vi "configure.vi"(8 "error in (no error)":errorcluster, 11 "DL090623TwoDAnalyser in":refnum<class "AnalyserDL090623TwoD.lvclass">) -> (0 "error out":errorcluster, 3 "DL090623TwoDAnalyser out":refnum<class "AnalyserDL090623TwoD.lvclass">)   [LabVIEW 2010, in "AnalyserDL090623TwoD.lvclass"]
doc: "The dynamic dispatch version of this VI loads and displays the configuration file associated with the plug-in object. The user modify and save the configuration data."
uses:
  AnalyserDL090623TwoD.lvclass
  common/xcontrols/XComponentSpecification/XComponentSpecification/XComponentSpecification.xctl
  AnalyserDL090623TwoD.lvclass/AnalyserDL090623TwoD.ctl
  Segmenter/GenericSegmenter/GenericSegmenter/GenericSegmenter.lvclass
  TraceProcessor/GenericTraceProcessor/GenericTraceProcessor/GenericTraceProcessor.lvclass
  common/classes/ErrorController/ErrorController/class_data.vi
  common/classes/GenericComponent/GenericComponent/GenericComponent.lvclass
  common/classes/ErrorController/ErrorController/ErrorController.lvclass
panel:
  in  "segmenter spec":T1(xcontrol)
  out "Configuration":string
  in  "Tab Control":T2(tab)
  in  "channel calculation expression":string
  in  "configure trace processors":bool
  in  "cancel button":bool
  in  "save button":bool
  # "Configure AnalyserDL090623TwoD"
  # "The AnalyserDL090623TwoD component receives images and calculates the mean signal intensity on image ROIs according to an arithmetic expression (see trace specification). \nROIs can either be drawn by hand and automatically determined using a Segmenter. \nThese intensity values are sent through a pipeline of TraceProcessors, which can perform further mathematic analysis on them."
  # "This mathematic term specifies how traces are calculated from channels. Enter an expression containing the channels as capital letters in alphabetic order. \nIMPORTANT: Numeric constants are not yet supported.\n\n \n- if you want to refer to the second channel only: B\n- if you want to refer to the ratio of the second and third channel: B/C\n- more complicated example: (A-B)/C+D"
  # "Traces calculated from the channels based on the trace specification expression given on the previous tab are processed by a user-defined pipeline of TraceProcessors. Each TraceProcessor may have a display to show its result."
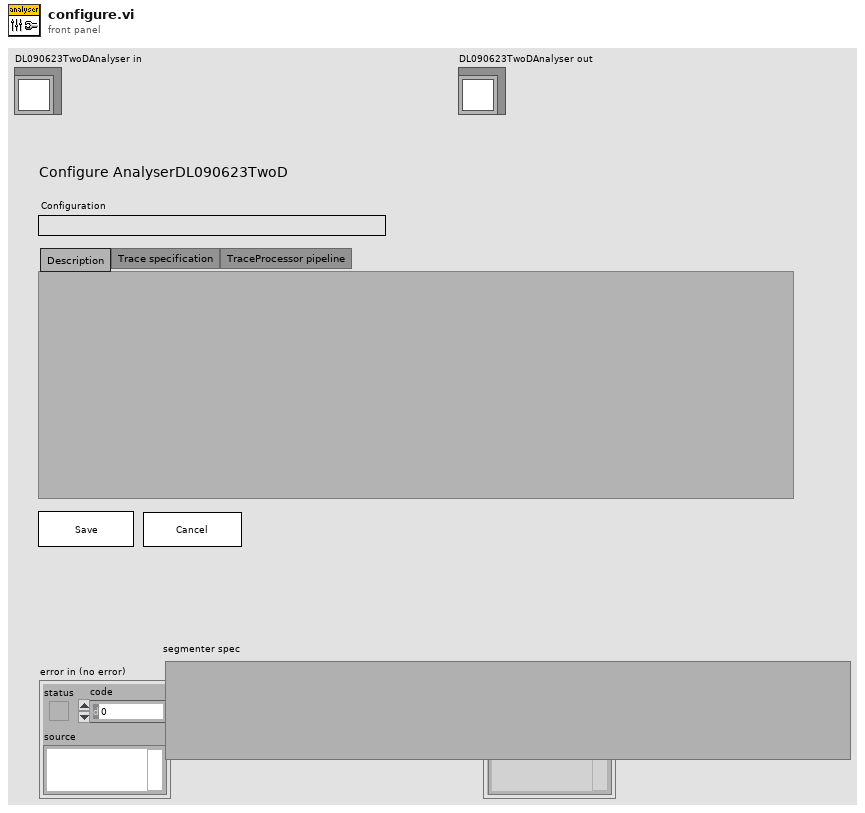
[diagram p1: front panel]
types:
  T1 = cluster{"class path":string, "configuration":string, "label":string, "settings name":string}
  T2 = enum32{"Description", "Trace specification", "TraceProcessor pipeline"}
  T3 = typedef "plugin_specification.ctl" = cluster{"class path":string, "configuration":string, "label":string, "settings name":string}
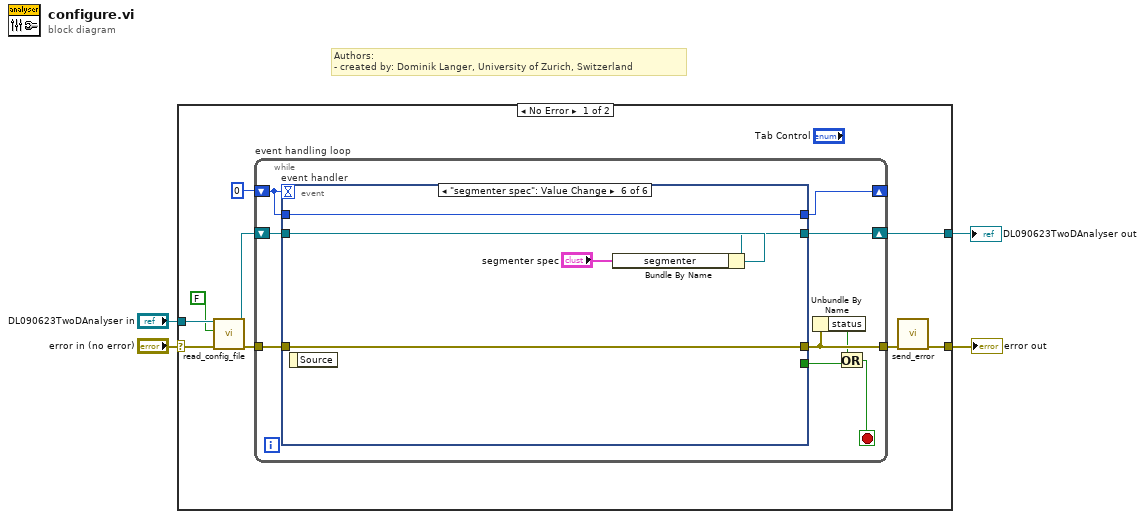
[diagram p0: block diagram]
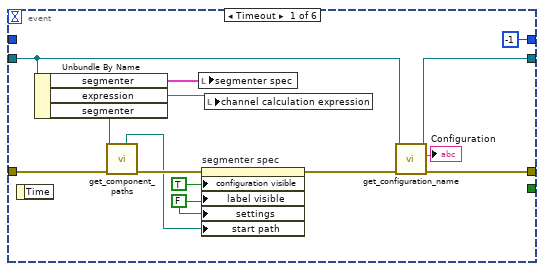
[diagram p2: hidden frame]
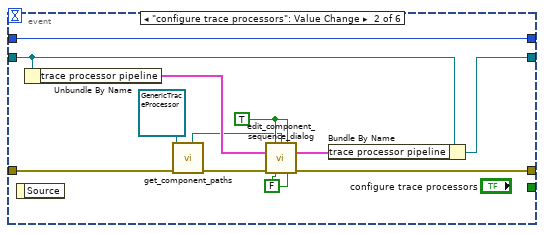
[diagram p3: hidden frame]
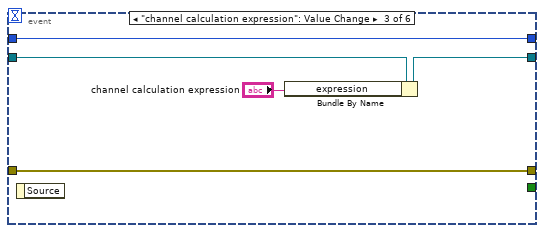
[diagram p4: hidden frame]
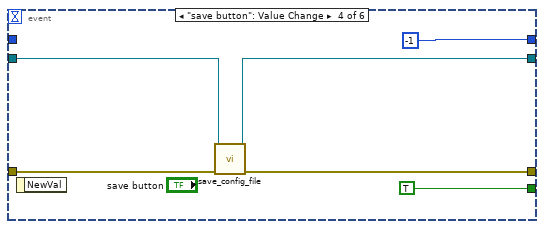
[diagram p5: hidden frame]
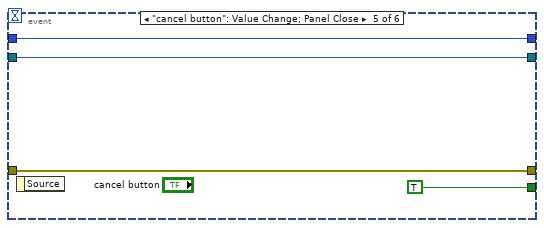
[diagram p6: hidden frame]
diagram:
  # "Authors: \n- created by: Dominik Langer, University of Zurich, Switzerland"
  n1 = case shown="No Error" "error in (no error)" {
    selector: "error in (no error)" -> [w11 w69]
    tunnel: [w7 w69] -> w3
    tunnel: "DL090623TwoDAnalyser in" -> [w9 w70]
    tunnel: [w13 w70] -> w1
    frame No Error {
      n2 = call-dynamic "read_config_file.vi"("error in (no error)"=w11, "force load?"=FALSE, "GenericPlugin in"=w9) -> ("error out"=w10:errorcluster, "GenericPlugin out"=w5:refnum<class "AnalyserDL090623TwoD.lvclass">)  [unwired: 7 out]
      n3 = while "event handling loop" {
        shift-right: [w20] -> w13
        shift-left: w5 -> [w21]
        shift-right: [w18] -> _
        shift-left: 0 -> [w19]
        tunnel: w10 -> [w22]
        tunnel: [w17] -> w6
        stop <- w14 stop-if-true
        n4 = event "event handler" shown="[5] \"segmenter spec\": Value Change" {
          selector: _ -> [_ _ _ _ _ _]
          dyn-events: _ -> [_ _ _ _ _ _]
          timeout: w19 -> [_ _ _ _ _ _]
          tunnel: w22 -> [w28 w41 w53 w59 w63 w64]
          tunnel: [w34 w47 w53 w58 w63 w64] -> w17
          tunnel: w21 -> [w33 w37 w51 w54 w62 w67]
          tunnel: [w32 w43 w50 w57 w62 w66] -> w20
          tunnel: [-1 w48 w52 -1 w61 w68] -> w18
          tunnel: w19 -> [_ w48 w52 _ w61 w68]
          tunnel: [_ _ _ TRUE TRUE _] -> w15
          event Timeout {
            w23 = FALSE ("label visible")
            n5 = event-data() -> ()  [unwired: 2 out]
            n6 = Unbundle By Name(w33) -> ("segmenter"=w30:T3, "expression"=w36:string, "segmenter"=w29:refnum<class "GenericSegmenter.lvclass">)
            n7 = call-dynamic "get_component_paths.vi"("error in (no error)"=w28, "GenericComponent in"=w29) -> ("error out"=w27:errorcluster, "component type directory"=w26:path)  [unwired: 4 in, 4 out]
            n8 = local write "segmenter spec"(w30) -> ()
            n9 = property on="segmenter spec" class="XComponentSpecification (strict"(error in=w27, "configuration visible"=TRUE, "label visible"=w23, "settings"=w23, "start path"=w26) -> (error out=w25:errorcluster)  [unwired: 1 in, 1 out]
            n10 = local write "channel calculation expression"(w36) -> ()
            n11 = call "get_configuration_name.vi"("error in (no error)"=w25, "GenericPlugin.lvclass in"=w33) -> ("error out"=w34:errorcluster, "configuration name"=→"Configuration":string, "GenericPlugin.lvclass out"=w32:refnum<class "AnalyserDL090623TwoD.lvclass">)  [unwired: 7 in]
          }
          event "configure trace processors": Value Change {
            w42 = FALSE ("choose default?")
            w46 = TRUE ("show label?")
            n12 = event-data() -> ()  [unwired: 2 out]
            n13 = Unbundle By Name(w37) -> ("trace processor pipeline"=w45:T3[])
            n14 = call-dynamic "get_component_paths.vi"("error in (no error)"=w41, "GenericComponent in"=refnum<class "GenericTraceProcessor.lvclass"> refnum ("GenericTraceProcessor.lvclass")) -> ("error out"=w40:errorcluster, "component type directory"=w38:path)  [unwired: 4 in, 4 out]
            n15 = call "edit_component_sequence_dialog.vi"("show configuration?"=w46, "default folder path"=w38, "show label?"=w46, "component specification list in"=w45, "error in (no error)"=w40, "choose default?"=w42, "show settings?"=w42) -> ("component specification list out"=w44:T3[], "error out"=w47:errorcluster)  [unwired: 6 in, 1 out]
            n16 = Bundle By Name(cluster=w37, "trace processor pipeline"=w44) -> (w43:refnum<class "AnalyserDL090623TwoD.lvclass">)
          }
          event "channel calculation expression": Value Change {
            n17 = event-data() -> ()  [unwired: 2 out]
            n18 = Bundle By Name(cluster=w51, "expression"="channel calculation expression") -> (w50:refnum<class "AnalyserDL090623TwoD.lvclass">)
          }
          event "save button": Value Change {
            n19 = event-data() -> ()  [unwired: 2 out]
            n20 = call-dynamic "save_config_file.vi"("error in (no error)"=w59, "GenericPlugin in"=w54) -> ("error out"=w58:errorcluster, "GenericPlugin out"=w57:refnum<class "AnalyserDL090623TwoD.lvclass">)  [unwired: 1 in, 7 out]
          }
          event "cancel button": Value Change; Panel Close {
            n21 = event-data() -> ()  [unwired: 2 out]
          }
          event "segmenter spec": Value Change {
            n22 = event-data() -> ()  [unwired: 2 out]
            n23 = Bundle By Name(cluster=w67, "segmenter"="segmenter spec") -> (w66:refnum<class "AnalyserDL090623TwoD.lvclass">)
          }
        }
        n24 = Unbundle By Name(w17) -> ("status"=w16:bool)
        n25 = Or(x=w16, y=w15) -> (x .or. y?=w14:bool)
      }
      n26 = call "send_error.vi"("error in (no error)"=w6) -> ("error out"=w7:errorcluster)  [unwired: 10 in]
    }
    frame Error {
    }
  }
  "error out" <- w3
  "DL090623TwoDAnalyser out" <- w1
